vi "Process Joystick Button Event.vi"(6 "State":u8, 9 "Button":u8, 10 "Player":T1) -> ()   [LabVIEW 2021, in "Main Controller Actor.lvclass"]
uses:
  Main Controller Actor.lvclass
  Ship/Ship.lvclass
  Control State/Control State.lvclass
  Globals.vi
  Player.ctl
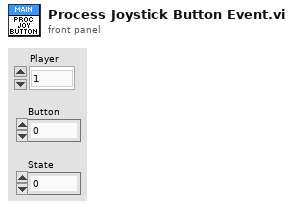
[diagram p1: front panel]
types:
  T1 = typedef "Main Controller Actor.lvclass/Player.ctl" = enum16{"1", "2"}
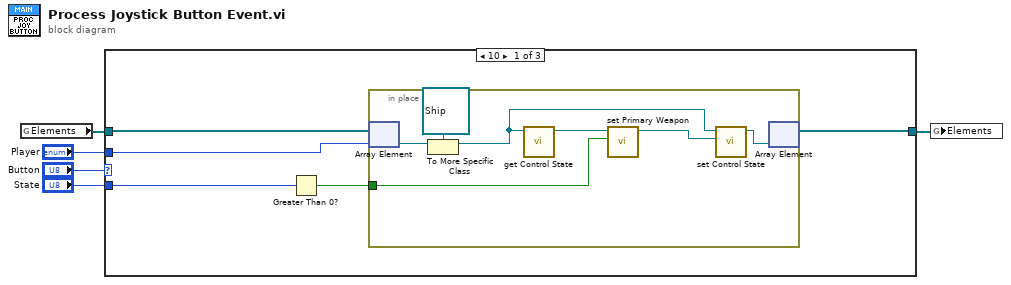
[diagram p0: block diagram]
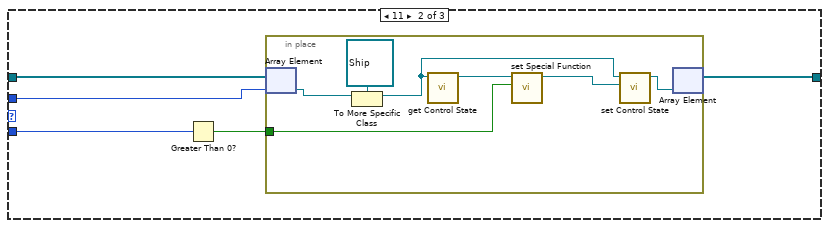
[diagram p2: hidden frame]
diagram:
  n1 = global read "Globals.vi" "Elements"() -> (w2:refnum<class "Element.lvclass">[])
  n2 = case shown="10" "Button" {
    tunnel: w2 -> [w7 w19 w30]
    tunnel: [w6 w18 w30] -> w1
    tunnel: "State" -> [w10 w22 _]
    tunnel: "Player" -> [w9 w21 _]
    frame 10 {
      n3 = Greater Than 0?(x=w10) -> (x > 0?=w8:bool)
      n4 = in-place {
        in-place-border: w8 -> [w15]
        n5 = in-place-array #1(w7, w9) -> (w12:refnum<class "Element.lvclass">)
        n6 = To More Specific Class(target class=refnum<class "Ship.lvclass"> refnum ("Ship in"), reference=w12) -> (specific class reference=w11:refnum<class "Ship.lvclass">)  [unwired: 1 in, 1 out]
        n7 = call "get Control State.vi"("Ship in"=w11) -> ("Control State"=w17:refnum<class "Control State.lvclass">)  [unwired: 10 in]
        n8 = call "set Primary Weapon.vi"("Primary Weapon"=w15, "Control State in"=w17) -> ("Control State out"=w16:refnum<class "Control State.lvclass">)  [unwired: 9 in]
        n9 = call-dynamic "set Control State.vi"("Control State"=w16, "Ship in"=w11) -> ("Ship out"=w14:refnum<class "Ship.lvclass">)  [unwired: 9 in]
        n10 = in-place-array #1(w14) -> (w6:refnum<class "Element.lvclass">[])  [unwired: 1 out]
      }
    }
    frame 11 {
      n11 = Greater Than 0?(x=w22) -> (x > 0?=w20:bool)
      n12 = in-place {
        in-place-border: w20 -> [w27]
        n13 = in-place-array #2(w19, w21) -> (w24:refnum<class "Element.lvclass">)
        n14 = To More Specific Class(target class=refnum<class "Ship.lvclass"> refnum ("Ship in"), reference=w24) -> (specific class reference=w23:refnum<class "Ship.lvclass">)  [unwired: 1 in, 1 out]
        n15 = call "get Control State.vi"("Ship in"=w23) -> ("Control State"=w29:refnum<class "Control State.lvclass">)  [unwired: 10 in]
        n16 = call "set Special Function.vi"("Special Function"=w27, "Control State in"=w29) -> ("Control State out"=w28:refnum<class "Control State.lvclass">)  [unwired: 9 in]
        n17 = call-dynamic "set Control State.vi"("Control State"=w28, "Ship in"=w23) -> ("Ship out"=w26:refnum<class "Ship.lvclass">)  [unwired: 9 in]
        n18 = in-place-array #2(w26) -> (w18:refnum<class "Element.lvclass">[])  [unwired: 1 out]
      }
    }
    frame Default {
    }
  }
  n19 = global write "Globals.vi" "Elements"(w1) -> ()
